vi "Service Location FGV Impl.vi"(6 "resolve service request":T2, 8 "error in":errorcluster, 9 "location unique id in":u64, 10 "action":T1, 11 "resolve vi reference":refnum<vi>) -> (0 "error out":errorcluster, 1 "location unique id out":u64, 2 "service location":T3)   [LabVIEW 2020, in "Plug-In SDK Discovery V1.lvlib"]
uses:
  Plug-In SDK Discovery V1.lvlib
  gRPC/Generated APIs/ni/measurementlink/discovery/v1/RPC Messages/ni_measurementlink_discovery_v1_ServiceLocation.ctl
  gRPC/Generated APIs/ni/measurementlink/discovery/v1/RPC Messages/ni_measurementlink_discovery_v1_ResolveServiceRequest.ctl
  TypeDefs/Service Location FGV Action.ctl
  TypeDefs/Service Location Map Value.ctl
  <vilib>/Utility/miscctls.llb/LVMapReplaceAction.ctl
  gRPC/Generated APIs/ni/measurementlink/discovery/v1/ni.measurementlink.discovery.v1.lvlib
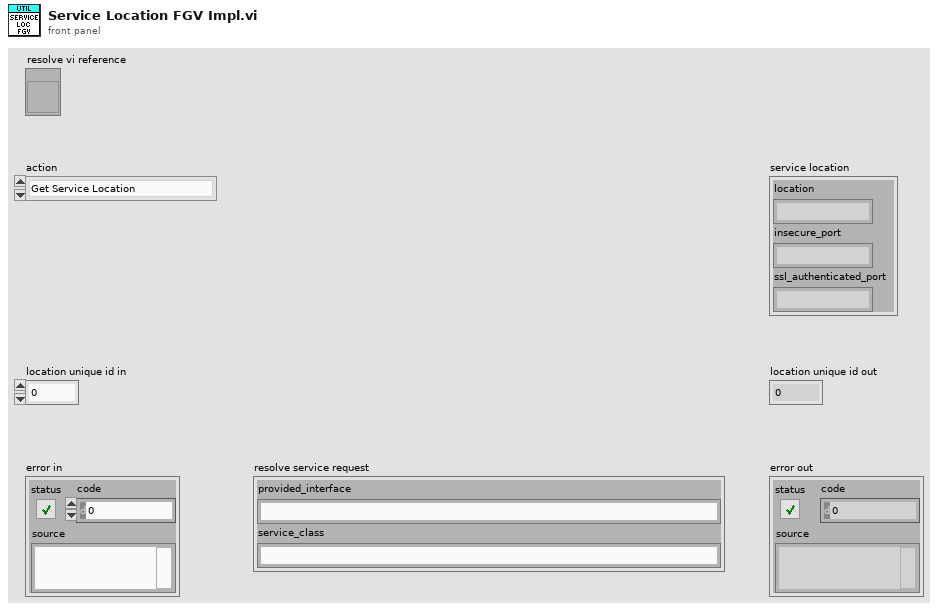
[diagram p1: front panel]
types:
  T1 = typedef "Plug-In SDK Discovery V1.lvlib/Service Location FGV Action.ctl" = enum16{"Get Service Location", "Reresolve Service Location"}
  T2 = typedef "ni.measurementlink.discovery.v1.lvlib/ni_measurementlink_discovery_v1_ResolveServiceRequest.ctl" = cluster{"provided_interface":string, "service_class":string}
  T3 = typedef "ni.measurementlink.discovery.v1.lvlib/ni_measurementlink_discovery_v1_ServiceLocation.ctl" = cluster{"location":string, "insecure_port":string, "ssl_authenticated_port":string}
  T4 = typedef "Plug-In SDK Discovery V1.lvlib/Service Location Map Value.ctl" = cluster{"response data":T3, "unique id":u64}
  T5 = typedef "LVMapReplaceAction.ctl" = enum32{"Modify Entry only if found", "Add or Modify Entry", "Delete Entry"}
  T6 = typedef "MeasurementLink Discovery Client.lvlib/ni_measurementlink_discovery_v1_ServiceLocation.ctl" = cluster{"location":string, "insecure_port":string, "ssl_authenticated_port":string}
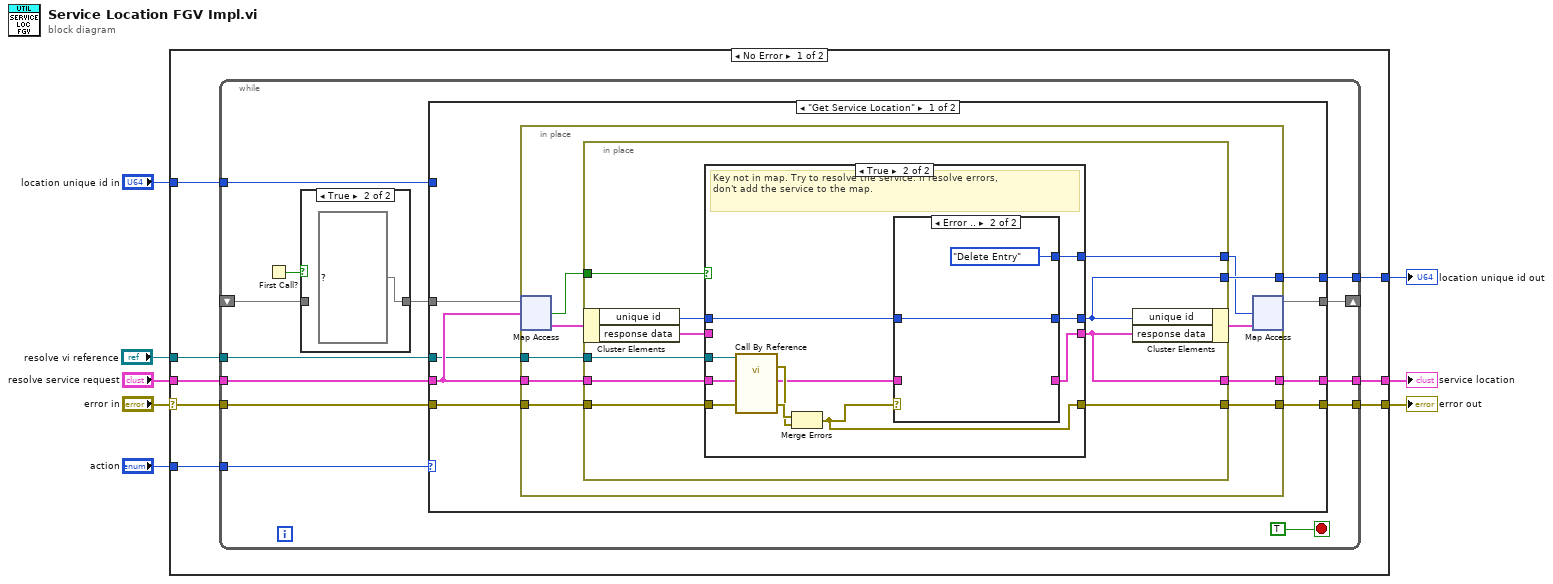
[diagram p0: block diagram]
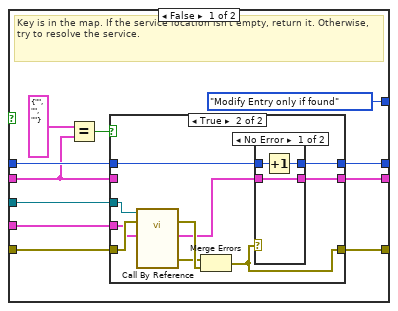
[diagram p3: hidden frame]
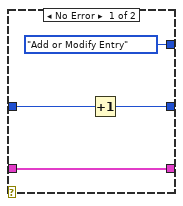
[diagram p6: hidden frame]
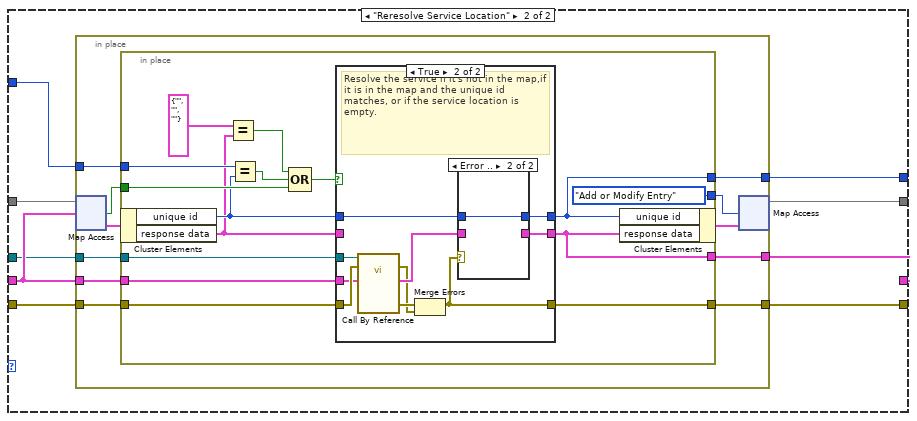
[diagram p7: hidden frame]
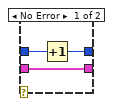
[diagram p9: hidden frame]
diagram:
  n1 = case shown="No Error" "error in" {
    selector: "error in" -> [w16 w157]
    tunnel: [w13 w157] -> w6
    tunnel: [w15 _] -> w8
    tunnel: "resolve service request" -> [w14 _]
    tunnel: "action" -> [w12 _]
    tunnel: [w11 _] -> w3
    tunnel: "location unique id in" -> [w10 _]
    tunnel: "resolve vi reference" -> [w9 _]
    frame No Error {
      n2 = while {
        shift-right: [w26] -> _
        shift-left: _ -> [w23]
        tunnel: w16 -> [w21]
        tunnel: [w28] -> w15
        tunnel: w14 -> [w27]
        tunnel: [w25] -> w13
        tunnel: w12 -> [w24]
        tunnel: [w19] -> w11
        tunnel: w10 -> [w18]
        tunnel: w9 -> [w17]
        stop <- TRUE stop-if-true
        n3 = First Call?() -> (First Call?: T/F=w20:bool)
        n4 = case shown="True" w20 {
          tunnel: w23 -> [w30 _]
          tunnel: [w30 map{T2, T4} {} ("map")] -> w22
          frame False {
          }
          frame True {
          }
        }
        n5 = case shown="\"Get Service Location\"" w24 {
          tunnel: w22 -> [w36 w113]
          tunnel: [w39 w107] -> w28
          tunnel: w27 -> [w34 w111]
          tunnel: w21 -> [w37 w110]
          tunnel: [w35 w108] -> w26
          tunnel: [w38 w109] -> w25
          tunnel: [w33 w106] -> w19
          tunnel: w18 -> [_ w112]
          tunnel: w17 -> [w32 w105]
          frame "Get Service Location" {
            n6 = in-place {
              in-place-border: w37 -> [w49]
              in-place-border: [w44] -> w39
              in-place-border: [w48] -> w38
              in-place-border: w34 -> [w46]
              in-place-border: [w45] -> w33
              in-place-border: w32 -> [w40]
              n7 = in-place-map #1(w36, w34) -> (w43:T4, w47:bool)  [unwired: 1 in]
              n8 = in-place {
                in-place-border: w49 -> [w59]
                in-place-border: [w58] -> w48
                in-place-border: w47 -> [w51]
                in-place-border: w46 -> [w57]
                in-place-border: [w55] -> w45
                in-place-border: [w54] -> w44
                in-place-border: [w53] -> w41
                in-place-border: w40 -> [w50]
                n9 = in-place-cluster #2(w43) -> ("unique id"=w56:u64, "response data"=w52:T3)
                n10 = case shown="True" w51 {
                  tunnel: w59 -> [w67 w92]
                  tunnel: [w66 w89] -> w58
                  tunnel: w57 -> [w64 w93]
                  tunnel: w56 -> [w63 w98]
                  tunnel: [w62 w97] -> w55
                  tunnel: w52 -> [w61 _]
                  tunnel: [w65 w96] -> w54
                  tunnel: [LVMapReplaceAction."Modify Entry only if found" ("action") w95] -> w53
                  tunnel: w50 -> [w60 w94]
                  frame False {
                    # "Key is in the map. If the service location isn't empty, return it. Otherwise, try to resolve the service."
                    n11 = Equal?(x=T3 {"location"="", "insecure_port"="", "ssl_authenticated_port"=""} ("y"), y=w61) -> (x = y?=w68:bool)
                    n12 = case shown="True" w68 {
                      tunnel: w67 -> [w73 w80]
                      tunnel: [w73 w76] -> w66
                      tunnel: [w71 w83] -> w65
                      tunnel: w64 -> [_ w75]
                      tunnel: w63 -> [w72 w82]
                      tunnel: [w72 w81] -> w62
                      tunnel: w61 -> [w71 _]
                      tunnel: w60 -> [_ w79]
                      frame False {
                      }
                      frame True {
                        n13 = call-by-ref "?"(reference=w79, error in=w80, "request data"=w75) -> (error out=w78:errorcluster, 0:"error out"=w77:errorcluster, "response data"=w74:T6)  [unwired: 9 in, 1 out]
                        n14 = Merge Errors(w77, w78) -> (w76:errorcluster)
                        n15 = case shown="No Error" w76 {
                          tunnel: [w84 _] -> w83
                          tunnel: w82 -> [w86 w87]
                          tunnel: [w85 w87] -> w81
                          tunnel: w74 -> [w84 _]
                          frame No Error {
                            n16 = Increment(x=w86) -> (x+1=w85:u64)
                          }
                          frame Error {
                          }
                        }
                      }
                    }
                  }
                  frame True {
                    # "Key not in map. Try to resolve the service. If resolve errors,\ndon't add the service to the map."
                    n17 = call-by-ref "?"(reference=w94, "error in"=w92, "request data"=w93) -> (error out=w90:errorcluster, 0:"error out"=w91:errorcluster, "response data"=w88:T6)  [unwired: 9 in, 1 out]
                    n18 = Merge Errors(w91, w90) -> (w89:errorcluster)
                    n19 = case shown="Error .." w89 {
                      tunnel: w98 -> [w102 w104]
                      tunnel: [w101 w104] -> w97
                      tunnel: w88 -> [w100 _]
                      tunnel: [w100 _] -> w96
                      tunnel: [LVMapReplaceAction."Add or Modify Entry" ("action") LVMapReplaceAction."Delete Entry" ("action")] -> w95
                      frame No Error {
                        n20 = Increment(x=w102) -> (x+1=w101:u64)
                      }
                      frame Error {
                      }
                    }
                  }
                }
                n21 = in-place-cluster #2("unique id"=w55, "response data"=w54) -> (w42:T4)
              }
              n22 = in-place-map #1(w42, w41) -> (w35:map{T2, T4})  [unwired: 2 out]
            }
          }
          frame "Reresolve Service Location" {
            n23 = in-place {
              in-place-border: w112 -> [w124]
              in-place-border: w111 -> [w122]
              in-place-border: w110 -> [w121]
              in-place-border: [w120] -> w109
              in-place-border: [w117] -> w107
              in-place-border: [w116] -> w106
              in-place-border: w105 -> [w114]
              n24 = in-place-map #3(w113, w111) -> (w119:T4, w123:bool)  [unwired: 1 in]
              n25 = in-place {
                in-place-border: w124 -> [w139]
                in-place-border: w123 -> [w133]
                in-place-border: w122 -> [w136]
                in-place-border: w121 -> [w135]
                in-place-border: [w134] -> w120
                in-place-border: [w132] -> w117
                in-place-border: [w130] -> w116
                in-place-border: [LVMapReplaceAction."Add or Modify Entry" ("action")] -> w115
                in-place-border: w114 -> [w125]
                n26 = in-place-cluster #4(w119) -> ("unique id"=w131:u64, "response data"=w128:T3)
                n27 = Equal?(x=T3 {"location"="", "insecure_port"="", "ssl_authenticated_port"=""} ("y"), y=w128) -> (x = y?=w126:bool)
                n28 = Equal?(x=w139, y=w131) -> (x = y?=w137:bool)
                n29 = Compound Arithmetic op=OR(w126, w137, w133) -> (w138:bool)
                n30 = case shown="True" w138 {
                  tunnel: w136 -> [_ w147]
                  tunnel: w135 -> [w142 w149]
                  tunnel: [w142 w144] -> w134
                  tunnel: [w140 w152] -> w132
                  tunnel: w131 -> [w141 w151]
                  tunnel: [w141 w150] -> w130
                  tunnel: w128 -> [w140 _]
                  tunnel: w125 -> [_ w148]
                  frame False {
                    # "The key is in the map and the unique id doesn't match, which means the service was already re-resolved."
                  }
                  frame True {
                    # "Resolve the service if it's not in the map,if it is in the map and the unique id matches, or if the service location is empty."
                    n31 = call-by-ref "?"(reference=w148, error in=w149, "request data"=w147) -> (error out=w143:errorcluster, 0:"error out"=w145:errorcluster, "response data"=w146:T6)  [unwired: 9 in, 1 out]
                    n32 = Merge Errors(w145, w143) -> (w144:errorcluster)
                    n33 = case shown="Error .." w144 {
                      tunnel: w146 -> [w155 _]
                      tunnel: [w155 _] -> w152
                      tunnel: w151 -> [w154 w156]
                      tunnel: [w153 w156] -> w150
                      frame No Error {
                        n34 = Increment(x=w154) -> (x+1=w153:u64)
                      }
                      frame Error {
                      }
                    }
                  }
                }
                n35 = in-place-cluster #4("unique id"=w130, "response data"=w132) -> (w118:T4)
              }
              n36 = in-place-map #3(w118, w115) -> (w108:map{T2, T4})  [unwired: 2 out]
            }
          }
        }
      }
    }
    frame Error {
    }
  }
  "error out" <- w6
  "service location" <- w8
  "location unique id out" <- w3
